vi "Chi Square Distribution.vi"(2 "degrees of freedom":i32=1 format="%0.0f", 3 "x":dbl format="%0.4f") -> (0 "error":i32, 1 "probability":dbl format="%0.4f")   [LabVIEW 2018, in "NI_AALPro.lvlib"]
doc: "LabVIEW no longer supports this VI. Use the Continuous CDF VI (Chi-Squared instance) instead. Computes the one-sided <B>probability</B>, p, of the distributed random variable, <B>x</B>, with the specified <B>degrees of freedom</B>. The Chi Square Distribution VI computes the one-sided <B>probability</B> such that the following condition is satisfied: p = Prob{X <= <B>x</B>}, where X is Chi squared distributed with n <B>degrees of freedom</B>, p is the <B>probability</B>, n is <B>degrees of freedom</B>, and <B>x</B> is the value."
uses:
  NI_AALPro.lvlib
  <resource>/lvanlys.dll
panel:
  # "Chi-Square Distribution"
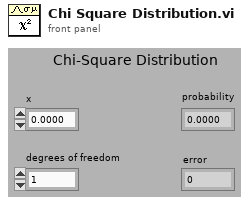
[diagram p1: front panel]
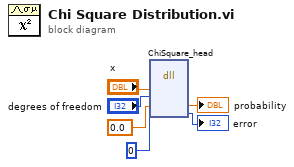
[diagram p0: block diagram]
diagram:
  n1 = dll-call lib="C:/Program Files (x86)/National Instruments/LabVIEW 2018/resource/lvanlys.*" fn="ChiSquare_head"("x"="x", "degrees of freedom"="degrees of freedom", 0.0, 0) -> (→"probability":dbl, →"error":i32)  [unwired: 6 in, 2 out]
